vi "FTW-Example-TransferClient.vi"() -> ()   [LabVIEW 2013]
uses:
  Windows/src/Transfer Client/dotNET/FTW-TransferClient-dotNET.lvclass
panel:
  in  "Local Destination Filepath":path=path "C:/Users/Jack/Desktop/test.txt"
  out "Current Rate (kB/sec)":dbl
  out "Iterations":i32
  out "AbsoluteURI":string
  out "Est. Time Remaining (sec)":dbl
  out "Cancelled?":bool
  out "Local Destination":path
  out "error out":errorcluster
  in  "Remote URI":string="ftp://ftp.ni.com/evaluation/labview/MotionAssistant250.exe"
  out "Total MB":dbl
  out "Error Message":string
  out "Error?":bool
  out "Percent Done":dbl(slide) scale=0.0..100.0
  in  "Cancel Download":bool
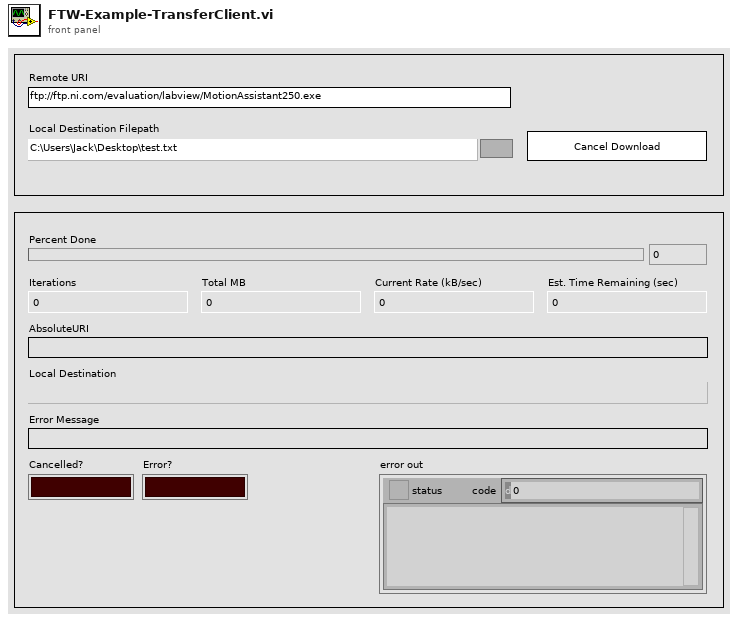
[diagram p1: front panel]
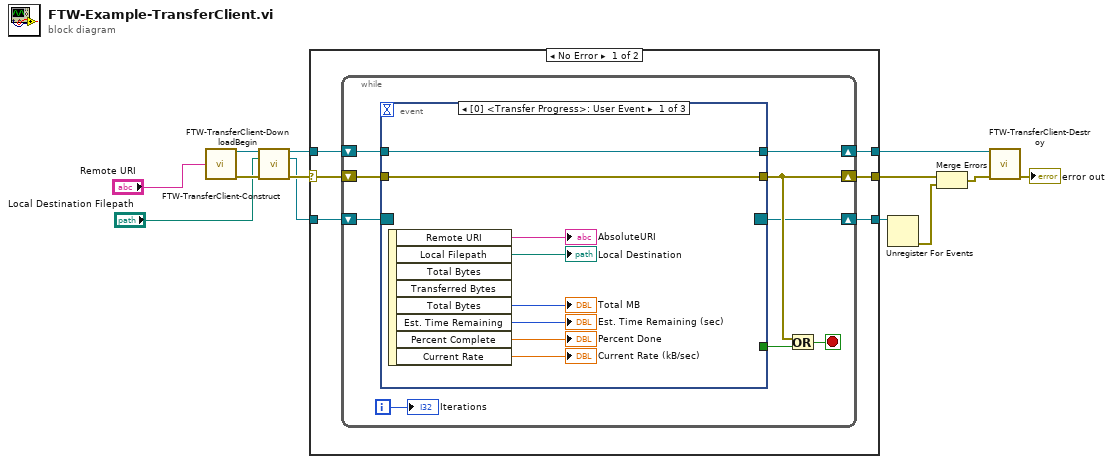
[diagram p0: block diagram]
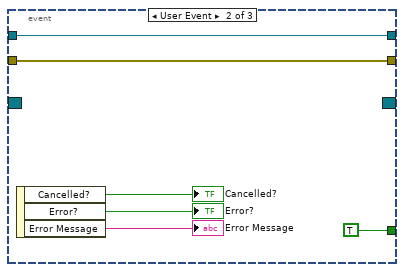
[diagram p2: hidden frame]
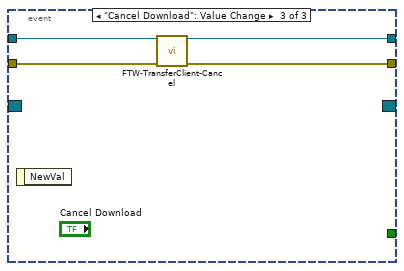
[diagram p3: hidden frame]
diagram:
  n1 = call "FTW-TransferClient-Construct.vi"("Remote URI"="Remote URI") -> ("Transfer Client"=w7:refnum<class "FTW-TransferClient-dotNET.lvclass">, "error out"=w5:errorcluster)  [unwired: 13 in]
  n2 = call-dynamic "FTW-TransferClient-DownloadBegin.vi"("TransferClient.dotNET"=w7, "Local Filepath"="Local Destination Filepath", "error in"=w5) -> ("TransferClient.dotNET out"=w6:refnum<class "FTW-TransferClient-dotNET.lvclass">, "Download Events"=w2:refnum<event-registration>, "error out"=w4:errorcluster)  [unwired: 10 in]
  n3 = case shown="No Error" w4 {
    selector: w4 -> [w16 w48]
    tunnel: w6 -> [w19 w49]
    tunnel: [w14 w47] -> w13
    tunnel: [w18 w49] -> w12
    tunnel: [w17 w48] -> w10
    tunnel: w2 -> [w15 w47]
    frame No Error {
      n4 = while {
        shift-right: [w26] -> w18
        shift-left: w19 -> [w28]
        shift-right: [w24] -> w17
        shift-left: w16 -> [w27]
        shift-right: [w20] -> w14
        shift-left: w15 -> [w21]
        i -> [w22]
        stop <- w23 stop-if-true
        n5 = event shown="[0] <Transfer Progress>: User Event" {
          selector: w21 -> [_ _ _]
          dyn-events: [_ _ _] -> w20
          timeout: _ -> [_ _ _]
          tunnel: w28 -> [w35 w40 w46]
          tunnel: [w34 w38 w44] -> w24
          tunnel: w27 -> [w34 w38 w45]
          tunnel: [w35 w40 w43] -> w26
          tunnel: [_ TRUE _] -> w25
          event User Event {
            n6 = event-data() -> ("Remote URI"=→"AbsoluteURI":string, "Local Filepath"=→"Local Destination":path, "Total Bytes"=→"Total MB":i64, "Est. Time Remaining"=→"Est. Time Remaining (sec)":u32, "Percent Complete"=→"Percent Done":dbl, "Current Rate"=→"Current Rate (kB/sec)":dbl)  [unwired: 1 in, 2 out]
          }
          event User Event {
            n7 = event-data() -> ("Cancelled?"=→"Cancelled?":bool, "Error?"=→"Error?":bool, "Error Message"=→"Error Message":string)  [unwired: 1 in]
          }
          event "Cancel Download": Value Change {
            n8 = event-data() -> ()  [unwired: 1 in, 1 out]
            n9 = call-dynamic "FTW-TransferClient-Cancel.vi"("TransferClient.dotNET"=w46, "error in"=w45) -> ("Transfer Client out"=w43:refnum<class "FTW-TransferClient-dotNET.lvclass">, "error out"=w44:errorcluster)  [unwired: 12 in]
          }
        }
        n10 = Or(x=w24, y=w25) -> (x .or. y?=w23:bool)
        "Iterations" <- w22
      }
    }
    frame Error {
    }
  }
  n11 = Unregister For Events(event registration refnum=w13) -> (error out=w9:errorcluster)  [unwired: 1 in]
  n12 = Merge Errors(w10, w9) -> (w8:errorcluster)
  n13 = call-dynamic "FTW-TransferClient-Destroy.vi"("TransferClient.dotNET"=w12, "error in"=w8) -> ("error out"=→"error out":errorcluster)  [unwired: 13 in]
